vi "Convert String to Engine.vi"(7 "transfer group id":i32, 8 "error in (no error)":errorcluster, 9 "string buffer":refnum<class "Buffer.lvclass">, 10 "engine buffer":refnum<class "Buffer.lvclass">, 11 "DSF Buffer Converter in":refnum<class "Default Buffer Converter.lvclass">) -> (0 "error out":errorcluster, 3 "DSF Buffer Converter out":refnum<class "Default Buffer Converter.lvclass">)   [LabVIEW 2017, in "DSF Core.lvlib" / "Default Buffer Converter.lvclass"]
uses:
  Default Buffer Converter.lvclass
  Classes/Buffer/Buffer.lvclass
  Default Buffer Converter.lvclass/Default Buffer Converter.ctl
  Move String Block.vi
  Classes/Buffer Converter/Convert String Data Type.vi
  VIs/Sizeof 1D.vi
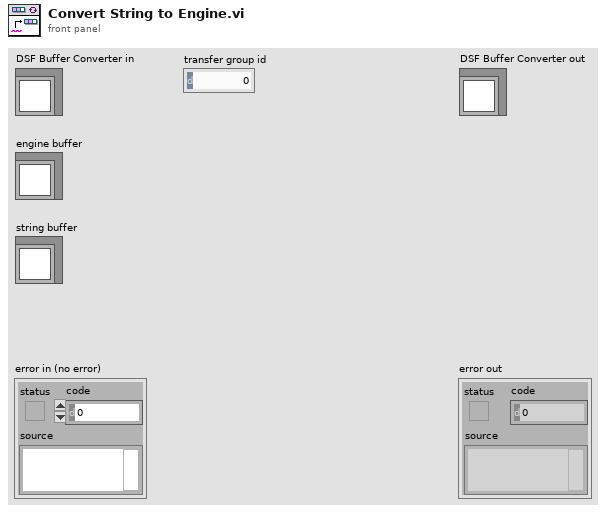
[diagram p1: front panel]
types:
  T1 = typedef "DSF Core.lvlib/Default Buffer Converter.lvclass/Conversion.ctl" = cluster{"conversion blocks":T2[]}
  T2 = typedef "DSF Core.lvlib/Default Buffer Converter.lvclass/Conversion Block.ctl" = cluster{"engine offset":u64, "engine data type":T3, "string offset":u64, "string data type":T3, "engine byte order":enum16{"big-endian, network order", "native, host order", "little-endian"}, "string byte order":enum16{"big-endian, network order", "native, host order", "little-endian"}, "count":u64}
  T3 = typedef "DSF Core.lvlib/DSF Data Type.ctl" = enum8{"Bool", "SGL", "DBL", "I8", "I16", "I32", "I64", "U8", "U16", "U32", "U64"}
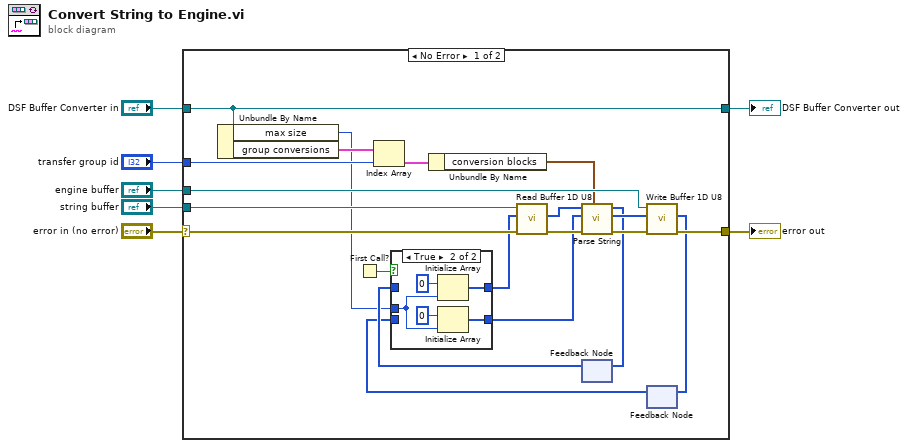
[diagram p0: block diagram]
diagram:
  n1 = case shown="No Error" "error in (no error)" {
    selector: "error in (no error)" -> [w13 w37]
    tunnel: [w12 w37] -> w6
    tunnel: [w26 w36] -> w4
    tunnel: "DSF Buffer Converter in" -> [w26 w36]
    tunnel: "transfer group id" -> [w25 _]
    tunnel: "string buffer" -> [w21 _]
    tunnel: "engine buffer" -> [w20 _]
    frame No Error {
      n2 = Unbundle By Name(w26) -> ("max size"=w8:u64, "group conversions"=w28:T1[])
      n3 = First Call?() -> (First Call?: T/F=w19:bool)
      n4 = Index Array(array=w28, index=w25) -> (element=w27:T1)
      n5 = Unbundle By Name(w27) -> ("conversion blocks"=w9:T2[])
      n6 = feedback #1() -> (w15:u8[])  [unwired: 1 in]
      n7 = feedback #2() -> (w14:u8[])  [unwired: 1 in]
      n8 = case shown="True" w19 {
        tunnel: w8 -> [_ w31]
        tunnel: [w29 w34] -> w11
        tunnel: [w30 w32] -> w18
        tunnel: w14 -> [w30 _]
        tunnel: w15 -> [w29 _]
        frame False {
        }
        frame True {
          n9 = Initialize Array(u8 0 ("element"), w31) -> (w34:u8[])
          n10 = Initialize Array(u8 0 ("element"), w31) -> (w32:u8[])
        }
      }
      n11 = call "Read Buffer 1D U8.vi"("error in (no error)"=w13, "dst array in"=w11, "Buffer in"=w21) -> ("error out"=w24:errorcluster, "dst array out"=w22:u8[])  [unwired: 5 in, 2 out]
      n12 = call "Parse String.vi"("conversion blocks"=w9, "error in (no error)"=w24, "engine buffer in"=w18, "string buffer in"=w22) -> ("error out"=w23:errorcluster, "engine buffer out"=w17:u8[], "string buffer out"=w16:u8[])  [unwired: 5 in]
      n13 = feedback-in #1(w16) -> ()
      n14 = call "Write Buffer 1D U8.vi"("error in (no error)"=w23, "src array in"=w17, "Buffer in"=w20) -> ("error out"=w12:errorcluster, "src array out"=w10:u8[])  [unwired: 5 in, 2 out]
      n15 = feedback-in #2(w10) -> ()
    }
    frame Error {
    }
  }
  "error out" <- w6
  "DSF Buffer Converter out" <- w4
